vi "Teleop.vi"(10 "Match Info":T1={"Autonomous Elapsed Seconds"=0.0, "TeleOp Elapsed Seconds"=0.0, "Disabled Elapsed Seconds"=0.0, "Visited Autonomous"=FALSE, "Visited TeleOp"=FALSE, "Visited Disabled"=FALSE, "Autonomous Settings"={"Autonomous Style"=enum."Independent", "VI Refnum"=refnum}}, 11 "Call Context":T2) -> ()   [LabVIEW 2014]
doc: "This VI is called for each TeleOp packet received from the DS where the robot is not disabled. It is often used to read from the joysticks and update I/O or to update setpoints for timed control loops. It should complete and return within 20 milliseconds or it may miss DS packets."
uses:
  <vilib>/Rock Robotics/WPI/DriverStation/WPI_DriverStationDerivedRobotMode.ctl
  <vilib>/Rock Robotics/WPI/DriverStation/WPI_DriverStationMatch Info.ctl
  <vilib>/Rock Robotics/Network Tables/SD Read Boolean.vi
panel:
  in  "AutoShift":bool
  in  "SecondaryRamping":dbl=0.2
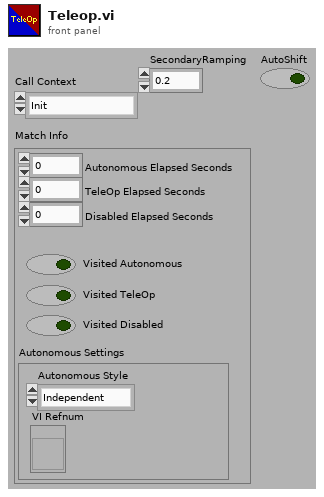
[diagram p1: front panel]
types:
  T1 = typedef "WPI_DriverStationMatch Info.ctl" = cluster{"Autonomous Elapsed Seconds":dbl, "TeleOp Elapsed Seconds":dbl, "Disabled Elapsed Seconds":dbl, "Visited Autonomous":bool, "Visited TeleOp":bool, "Visited Disabled":bool, "Autonomous Settings":cluster{"Autonomous Style":enum16{"Iterative", "Independent"}, "VI Refnum":refnum<vi>}}
  T2 = typedef "WPI_DriverStationDerivedRobotMode.ctl" = enum16{"Init", "Execute", "Stop"}
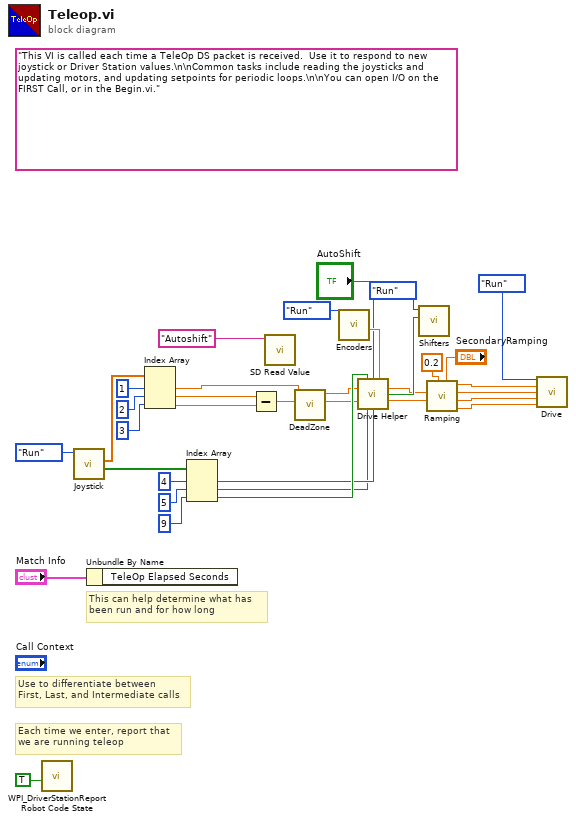
[diagram p0: block diagram]
diagram:
  (unwired) "This VI is called each time a TeleOp DS packet is received.  Use it to respond to new joystick or Driver Station values.\n\nCommon tasks include reading the joysticks and updating motors, and updating setpoints for periodic loops.\n\nYou can open I/O on the FIRST Call, or in the Begin.vi."
  # "Each time we enter, report that\nwe are running teleop"
  # "Use to differentiate between\nFirst, Last, and Intermediate calls"
  # "This can help determine what has\nbeen run and for how long"
  n1 = call <vilib>:"WPI_DriverStationReport Robot Code State.vi"("TeleOp"=TRUE ("Autonomous")) -> ()  [unwired: 10 in, 1 out]
  n2 = call "Joystick.vi"("Enum"=enum16{"Start", "Run", "End"}."Run") -> ("Buttons"=w26:bool[], "Axes"=w32:dbl[])  [unwired: 9 in]
  n3 = Unbundle By Name("Match Info") -> ()  [unwired: 1 out]
  n4 = Index Array(array=w32, index #1=1 ("index"), index #2=2 ("index"), index #3=3 ("index")) -> (element #1=w3:dbl, element #2=w28:dbl, element #3=w27:dbl)
  n5 = Index Array(array=w26, index #1=4 ("index"), index #2=5 ("index"), index #3=9 ("index")) -> (element #1=w21:bool, element #2=w20:bool, element #3=w22:bool)
  n6 = Subtract(x=w28, y=w27) -> (x-y=w4:dbl)
  n7 = call-poly <vilib>:"SD Read Value.vi"("Name"="Autoshift") -> ()  [unwired: 8 in, 3 out]
  n8 = call "DeadZone.vi"("Turn"=w4, "Speed"=w3) -> ("Turn  Out"=w2:dbl, "Speed Out"=w1:dbl)  [unwired: 8 in]
  n9 = call "Encoders.vi"("Enum"=enum16{"Start", "Run", "End"}."Run") -> ("Linear Speed"=w17:dbl)  [unwired: 7 in, 3 out]
  n10 = call "Drive Helper.vi"("QuickTurn"=w22, "AutoShift"="AutoShift", "Wheel Speed"=w17, "Throttle"=w1, "Turn"=w2, "ForceHigh"=w20, "ForceLow"=w21) -> ("Left Output"=w13:dbl, "isHighGear"=w15:bool, "Right Output"=w12:dbl)  [unwired: 6 in]
  n11 = call "Shifters.vi"("isHigh"=w15, "Enum"=enum16{"Start", "Run", "End"}."Run") -> ()  [unwired: 10 in]
  n12 = call "Ramping.vi"("SecondaryRamping"="SecondaryRamping", "PrimaryRamping"=0.2, "Right Power"=w12, "Left Power"=w13) -> ("Right Secondary"=w8:dbl, "Right Primary"=w9:dbl, "Left Secondary"=w10:dbl, "Left Primary"=w11:dbl)  [unwired: 4 in]
  n13 = call "Drive.vi"("Enum"=enum16{"Start", "Run", "End"}."Run", "Left Primary"=w11, "Left Secondary"=w10, "Right Primary"=w9, "Right Secondary"=w8) -> ()  [unwired: 11 in]
